vi "Default - Error.vi"(0 "object in":refnum<class "Document.lvclass">, 5 "error in (no error)":errorcluster) -> (14 "object out":refnum<class "Document.lvclass">, 19 "error out":errorcluster)   [LabVIEW 2014, in "Document.lvclass"]
uses:
  Document.lvclass
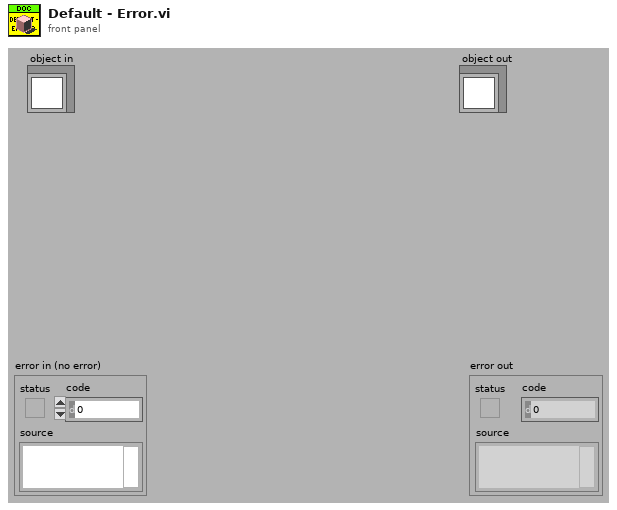
[diagram p1: front panel]
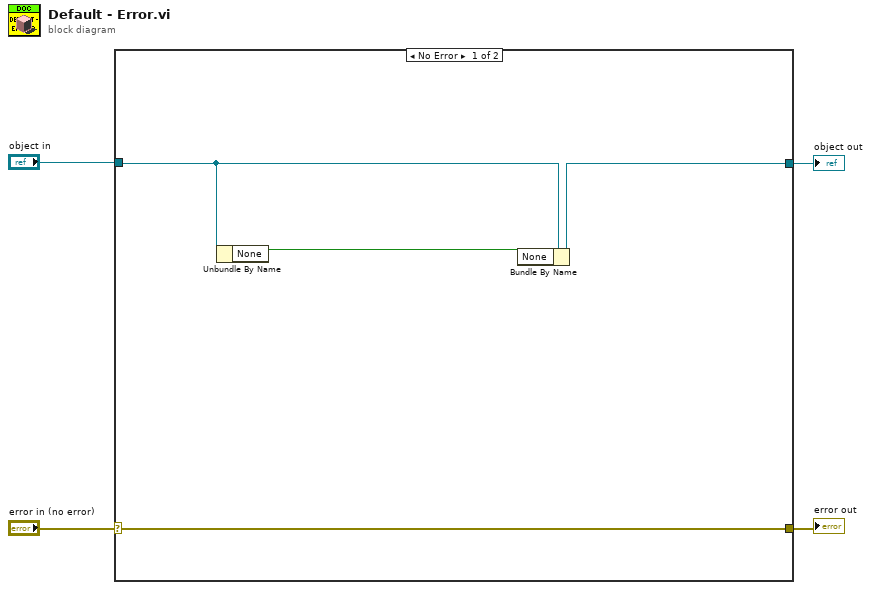
[diagram p0: block diagram]
diagram:
  n1 = case shown="No Error" "error in (no error)" {
    selector: "error in (no error)" -> [w7 w10]
    tunnel: [w7 w10] -> w3
    tunnel: [w5 w9] -> w1
    tunnel: "object in" -> [w6 w9]
    frame No Error {
      n2 = Unbundle By Name(w6) -> ("None"=w8:bool)
      n3 = Bundle By Name(cluster=w6, "None"=w8) -> (w5:refnum<class "Document.lvclass">)
    }
    frame Error {
    }
  }
  "error out" <- w3
  "object out" <- w1
